vi "Narrow+band+FM.vi"() -> ()   [LabVIEW 2011]
uses:
  <vilib>/measure/maspectr.llb/FFT Spectrum (Mag-Phase) for N Chan.vi
  <vilib>/measure/NI_MABase.lvlib
  <vilib>/Analysis/NI_AALBase.lvlib
  <vilib>/measure/NI_MAPro.lvlib
panel:
  out "signal out 6":dynamicdata(graph)
  out "Original":waveform(dbl)(graph)
  out "spectrum":cluster{"f0":dbl, "df":dbl, "magnitude":dbl[]}[](graph)
  out "signal out 5":dynamicdata(graph)
  out "filtered":dynamicdata(graph)
  out "FM out":dynamicdata(graph)
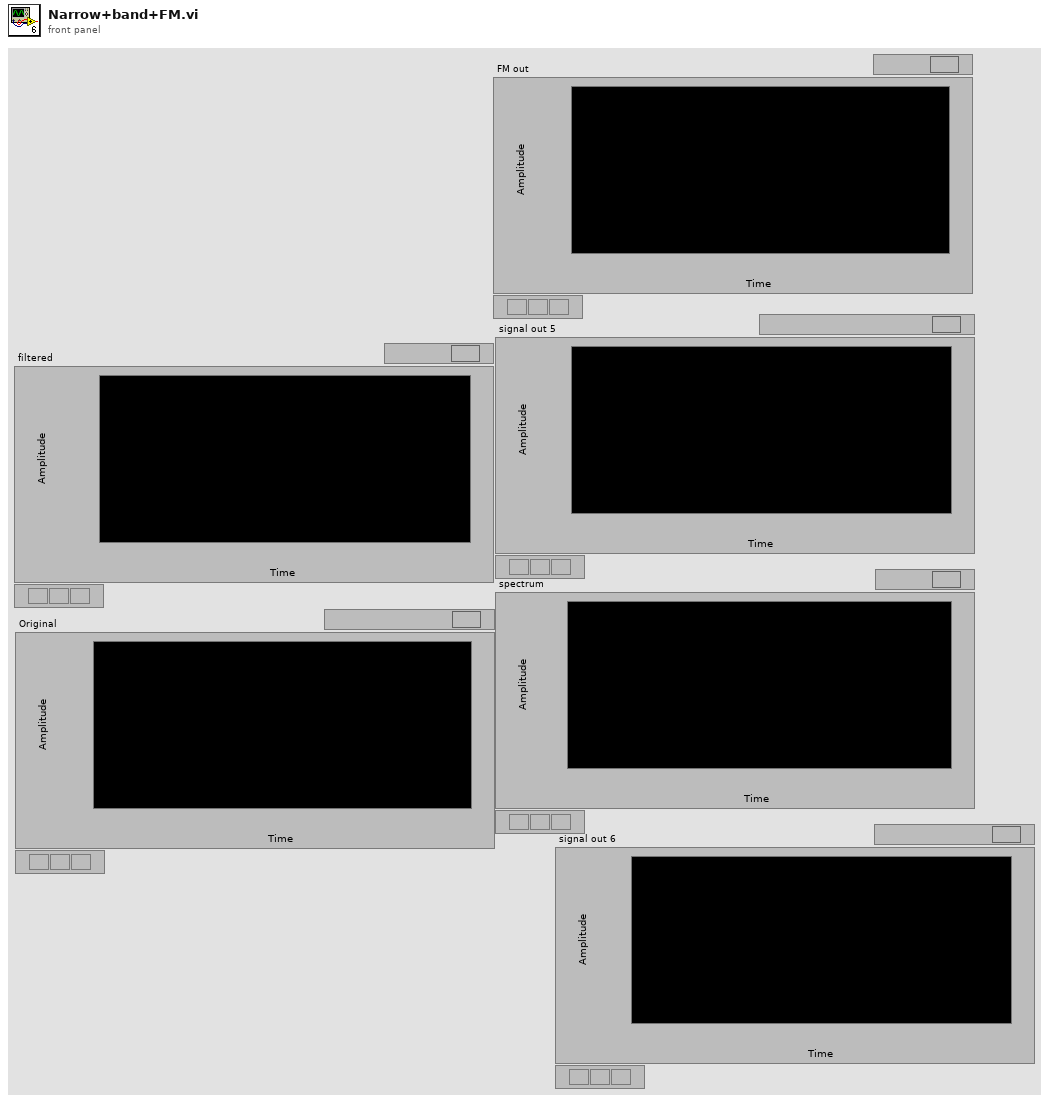
[diagram p1: front panel]
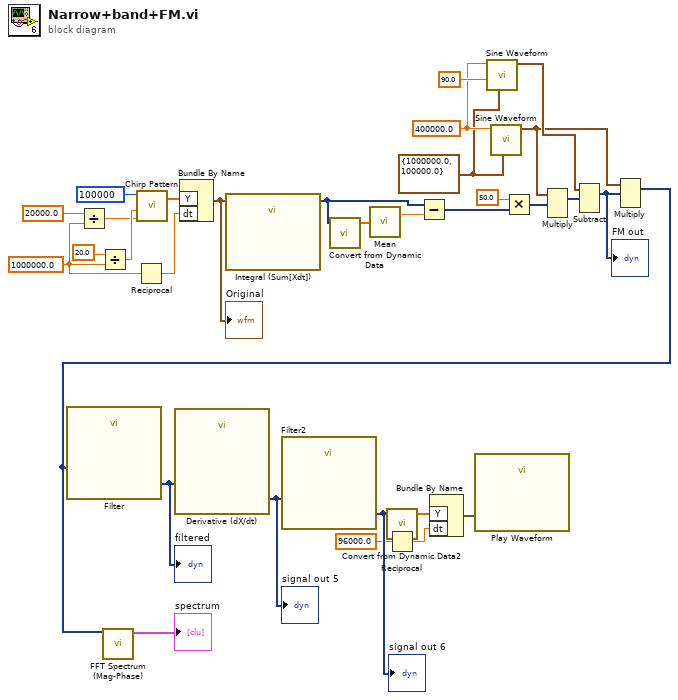
[diagram p0: block diagram]
diagram:
  w12 = 1000000.0 ("phase")
  w19 = cluster{"Fs":dbl, "#s":dbl} {"Fs"=1000000.0, "#s"=100000.0} ("sampling info")
  w25 = 400000.0 ("frequency")
  n1 = Divide(x=20000.0 ("phase"), y=w12) -> (x/y=w15:dbl)
  n2 = Divide(x=20.0 ("frequency"), y=w12) -> (x/y=w17:dbl)
  n3 = Reciprocal(x=w12) -> (1/x=w13:dbl)
  n4 = call <vilib>:"Chirp Pattern.vi"("f2"=w15, "f1"=w17, "samples"=100000) -> ("Chirp Pattern"=w14:dbl[])  [unwired: 1 in, 1 out]
  n5 = Bundle By Name("Y"=w14, "dt"=w13) -> (w11:waveform(dbl))  [unwired: 1 in]
  "Original" <- w11
  n6 = call "Integral (Sum[Xdt])"("Signals"=w11) -> ("Result"=w29:dynamicdata)  [unwired: 5 in, 1 out]
  n7 = call "Convert from Dynamic Data"("Dynamic Data Type"=w29) -> ("Array"=w28:dbl[])  [unwired: 3 in]
  n8 = call <vilib>:"Mean.vi"("X"=w28) -> ("mean"=w30:dbl)  [unwired: 1 out]
  n9 = Reciprocal(x=96000.0) -> (1/x=w3:dbl)
  n10 = Subtract(x=w29, y=w30) -> (x-y=w27:dynamicdata)
  n11 = call <vilib>:"Sine Waveform.vi"("sampling info"=w19, "phase"=90.0, "frequency"=w25) -> ("signal out"=w24:waveform(dbl))  [unwired: 7 in, 1 out]
  n12 = call <vilib>:"Sine Waveform.vi"("sampling info"=w19, "frequency"=w25) -> ("signal out"=w21:waveform(dbl))  [unwired: 8 in, 1 out]
  n13 = Multiply(x=50.0, y=w27) -> (x*y=w10:dynamicdata)
  n14 = Multiply(1:w10, 2:w21) -> (0:w23:dynamicdata)  [unwired: 1 in, 1 out]
  n15 = Subtract(1:w23, 2:w24) -> (0:w20:dynamicdata)  [unwired: 1 in, 1 out]
  "FM out" <- w20
  n16 = Multiply(1:w20, 2:w21) -> (0:w6:dynamicdata)  [unwired: 1 in, 1 out]
  n17 = call "Filter"("Signal"=w6) -> ("Filtered Signal"=w7:dynamicdata)  [unwired: 9 in, 1 out]
  "filtered" <- w7
  n18 = call-poly <vilib>:"FFT Spectrum (Mag-Phase).vi"("time signals"=w6) -> ("magnitudes"=→"spectrum":cluster{"f0":dbl, "df":dbl, "magnitude":dbl[]}[])  [unwired: 6 in, 4 out]
  n19 = call "Derivative (dX/dt)"("Signals"=w7) -> ("Result"=w8:dynamicdata)  [unwired: 5 in, 1 out]
  "signal out 5" <- w8
  n20 = call "Filter2"("Signal"=w8) -> ("Filtered Signal"=w5:dynamicdata)  [unwired: 9 in, 1 out]
  "signal out 6" <- w5
  n21 = call "Convert from Dynamic Data2"("Dynamic Data Type"=w5) -> ("Array"=w4:dbl[])  [unwired: 3 in]
  n22 = Bundle By Name("Y"=w4, "dt"=w3) -> (w1:waveform(dbl))  [unwired: 1 in]
  n23 = call "Play Waveform"("Data"=w1) -> ()  [unwired: 18 in, 1 out]
